vi "DP-Init StimGen.vi"(0 "Stimulus":T2={"Ear"=enum."Left", "f2 freqs (kHz)"="", "Start (dB)"=20.0, "Stop (dB)"=80.0, "Step (dB)"=10.0, "Mode"=enum."L1 = L2", "override recal"=FALSE, "Sampling Rate (Hz)"=0.0, "Frame (ms)"=0.0}, 11 "error in (no error)":errorcluster) -> (6 "DP Freqs":T1[](array[typedef]), 15 "error out":errorcluster)   [LabVIEW 2020]
uses:
  Typedefs/DP-Stimulus Params.ctl
  Typedefs/DP-Freqs.ctl
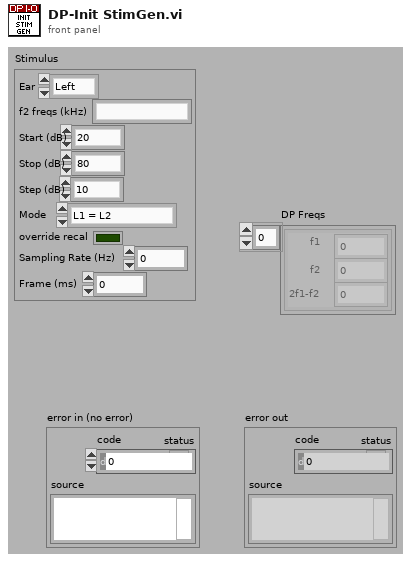
[diagram p1: front panel]
types:
  T1 = typedef "DP-Freqs.ctl" = cluster{"f1":dbl, "f2":dbl, "2f1-f2":dbl}
  T2 = typedef "DP-Stimulus Params.ctl" = cluster{"Ear":enum16{"Right", "Left"}, "f2 freqs (kHz)":string, "Start (dB)":dbl, "Stop (dB)":dbl, "Step (dB)":dbl, "Mode":enum16{"L1 = L2", "L1 = L2 + 10 dB"}, "override recal":bool, "Sampling Rate (Hz)":dbl, "Frame (ms)":dbl}
  T3 = cluster{"Coerced Frequency (kHz)":dbl, "Coerced Frequency (kHz)":dbl, dbl}
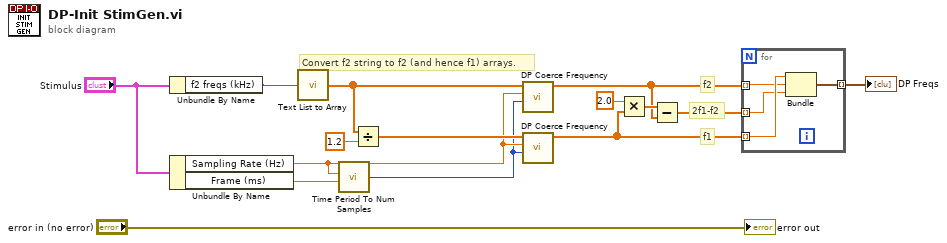
[diagram p0: block diagram]
diagram:
  # "2f1-f2"
  # "f2"
  # "f1"
  # "Convert f2 string to f2 (and hence f1) arrays."
  n1 = Unbundle By Name("Stimulus") -> ("f2 freqs (kHz)"=w14:string)
  n2 = Unbundle By Name("Stimulus") -> ("Sampling Rate (Hz)"=w2:dbl, "Frame (ms)"=w3:dbl)
  n3 = call "Text List to Array.vi"("text list"=w14) -> ("array"=w13:dbl[])  [unwired: 3 in]
  n4 = call "Time Period To Num Samples.vi"("Duration (ms)"=w2, "Sampling rate (Hz)"=w3) -> ("Samples"=w1:i32)  [unwired: 5 in]
  n5 = Divide(x=w13, y=1.2) -> (x/y=w12:dbl[])
  n6 = call "DP Coerce Frequency.vi"("Npts"=w1, "Sampling rate (Hz)"=w2, "Frequency (kHz)"=w13) -> ("Coerced Frequency (kHz)"=w10:dbl[])  [unwired: 6 in, 2 out]
  n7 = call "DP Coerce Frequency.vi"("Npts"=w1, "Sampling rate (Hz)"=w2, "Frequency (kHz)"=w12) -> ("Coerced Frequency (kHz)"=w8:dbl[])  [unwired: 6 in, 2 out]
  n8 = Multiply(x=2.0 ("y"), y=w8) -> (x*y=w11:dbl[])
  n9 = Subtract(x=w11, y=w10) -> (x-y=w7:dbl[])
  n10 = for {
    tunnel: w10 -> [w18] mode=indexing
    tunnel: w8 -> [w19] mode=indexing
    tunnel: w7 -> [w17] mode=indexing
    tunnel: [w16] -> w6 mode=indexing
    n11 = Bundle("Coerced Frequency (kHz)"=w19, "Coerced Frequency (kHz)"=w18, w17) -> (w16:T3)  [unwired: 1 in]
  }
  "DP Freqs" <- w6
  "error out" <- "error in (no error)"
